vi "mod_Calculate AWGN sample duration.vi"(0 "profile length (samples)":i32=1000, 5 "doppler filter taps":dbl[](array[numeric]) format="%.2f", 7 "interpolating filter taps":dbl[](array[numeric]) format="%.2f", 9 "interpolation factor":i32=1, 11 "error in (no error)":errorcluster, 13 "reset? (T)":bool=TRUE) -> (4 "AWGN samples":i32, 15 "error out":errorcluster)   [LabVIEW 2020, in "niDMT.lvlib"]
uses:
  <vilib>/addons/Modulation/niDMT.lvlib
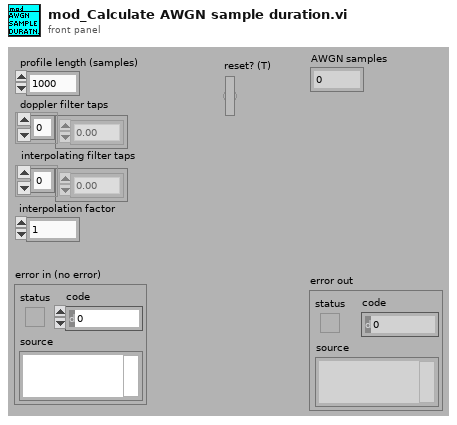
[diagram p1: front panel]
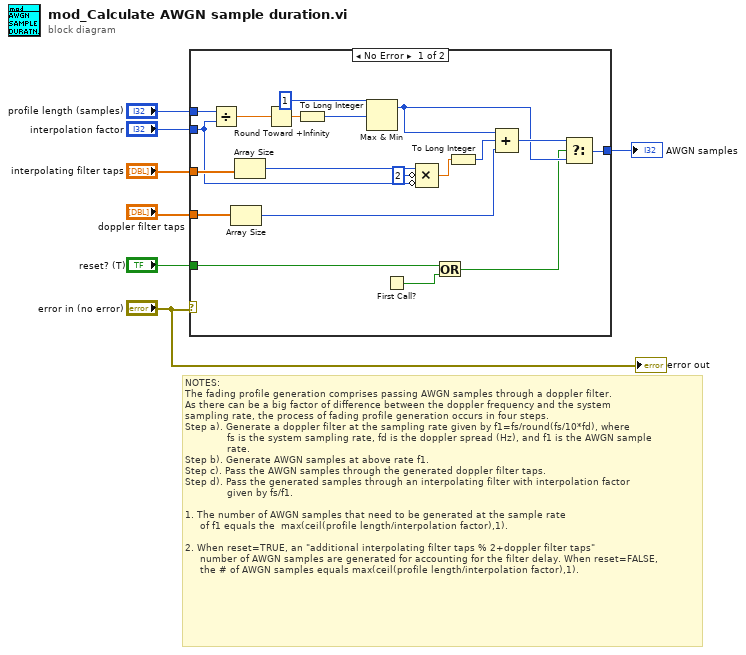
[diagram p0: block diagram]
diagram:
  # "NOTES:\nThe fading profile generation comprises passing AWGN samples through a doppler filter.\nAs there can be a big factor of difference between the doppler frequency and the system \nsampling rate, the process of fading profile generation occurs in four steps.\nStep a). Generate a doppler filter at the sampling rate given by f1=fs/round(fs/10*fd), where\n              fs is the system sampling rate, fd is the doppler spread (Hz), and f1 is the AWGN sample\n              rate.\nStep b). Generate AWGN samples at above rate f1.\nStep c). Pass the AWGN samples through the generated doppler filter taps.\nStep d). Pass the generated samples through an interpolating filter with interpolation factor\n              given by fs/f1.\n\n1. The number of AWGN samples that need to be generated at the sample rate\n     of f1 equals the  max(ceil(profile length/interpolation factor),1).\n\n2. When reset=TRUE, an \"additional interpolating filter taps % 2+doppler filter taps\" \n     number of AWGN samples are generated for accounting for the filter delay. When reset=FALSE,\n     the # of AWGN samples equals max(ceil(profile length/interpolation factor),1)."
  n1 = case shown="No Error" "error in (no error)" {
    tunnel: [w18 _] -> w7
    tunnel: "profile length (samples)" -> [w17 _]
    tunnel: "interpolation factor" -> [w10 _]
    tunnel: "reset? (T)" -> [w16 _]
    tunnel: "interpolating filter taps" -> [w15 _]
    tunnel: "doppler filter taps" -> [w14 _]
    frame No Error {
      n2 = Divide(x=w17, y=w10) -> (x/y=w24:dbl)
      n3 = Array Size(array=w14) -> (size(s)=w13:i32)
      n4 = Array Size(array=w15) -> (size(s)=w12:i32)
      n5 = Round Toward +Infinity(x=w24) -> (ceil(x): smallest int >= x=w21:dbl)
      n6 = To Long Integer(number=w21) -> (32bit integer=w25:i32)
      n7 = Max & Min(x=1, y=w25) -> (max(x,y)=w22:i32)  [unwired: 1 out]
      n8 = First Call?() -> (First Call?: T/F=w20:bool)
      n9 = Compound Arithmetic op=MULTIPLY(w12, invert 2 ("value"), invert w10) -> (w9:dbl)
      n10 = Or(x=w16, y=w20) -> (x .or. y?=w19:bool)
      n11 = To Long Integer(number=w9) -> (32bit integer=w8:i32)
      n12 = Compound Arithmetic op=ADD(w22, w8, w13) -> (w26:i32)
      n13 = Select(t=w26, s=w19, f=w22) -> (s? t:f=w18:i32)
    }
    frame Error {
    }
  }
  "AWGN samples" <- w7
  "error out" <- "error in (no error)"
